vi "IntakeDefaultControl.vi"(10 "On":bool) -> ()   [LabVIEW 2014, in "IntakeLib.lvlib"]
uses:
  IntakeLib.lvlib
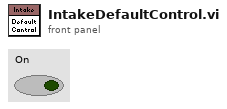
[diagram p1: front panel]
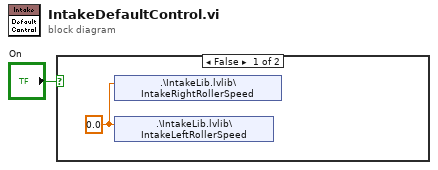
[diagram p0: block diagram]
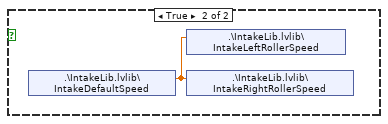
[diagram p2: hidden frame]
diagram:
  n1 = case shown="False" "On" {
    frame False {
      w2 = 0.0 ("IntakeLeftRollerSpeed")
      n2 = shared-variable ".\\IntakeLib.lvlib\\IntakeRightRollerSpeed"(w2) -> ()  [unwired: 1 in, 1 out]
      n3 = shared-variable ".\\IntakeLib.lvlib\\IntakeLeftRollerSpeed"(w2) -> ()  [unwired: 1 in, 1 out]
    }
    frame True {
      n4 = shared-variable ".\\IntakeLib.lvlib\\IntakeDefaultSpeed"() -> (w3:dbl)  [unwired: 1 in, 1 out]
      n5 = shared-variable ".\\IntakeLib.lvlib\\IntakeLeftRollerSpeed"(w3) -> ()  [unwired: 1 in, 1 out]
      n6 = shared-variable ".\\IntakeLib.lvlib\\IntakeRightRollerSpeed"(w3) -> ()  [unwired: 1 in, 1 out]
    }
  }
